vi "TDMS Delete NULL Strings from array.vi"(11 "String Array":string[](array[string])) -> (3 "String Array w/o NULL":string[](array[string]))   [LabVIEW 2011]
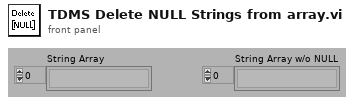
[diagram p1: front panel]
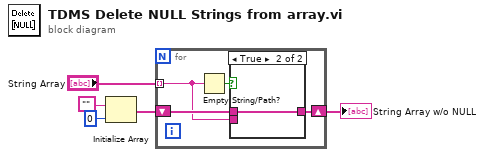
[diagram p0: block diagram]
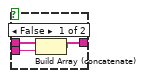
[diagram p2: hidden frame]
diagram:
  n1 = Initialize Array("", 0 ("dimension size")) -> (w2:string[])
  n2 = for {
    tunnel: "String Array" -> [w6] mode=indexing
    shift-right: [w7] -> w5
    shift-left: w2 -> [w8]
    n3 = Empty String/Path?(string/path=w6) -> (empty?=w9:bool)
    n4 = case shown="True" w9 {
      tunnel: w8 -> [w11 w13]
      tunnel: [w12 w13] -> w7
      tunnel: w6 -> [w10 _]
      frame False {
        n5 = Build Array (concatenate)(w11, w10) -> (w12:string[])
      }
      frame True {
      }
    }
  }
  "String Array w/o NULL" <- w5
